vi "FGEN_OPEN.vi"(8 "error in":errorcluster caption="error in (no error)", 10 "channel parameters":T3(array[cluster])=[{"channel name"="0", "waveform"=5, "frequency"=1000000.0, "amplitude"=1.0, "start phase"=0.0, "dc offset"=-0.05, "duty cycle high"=50.0, "impedance"=0, "load impedance"=-1.0}] {"waveform" items=["Sine", "Square", "Triangle", "Ramp Up", "Ramp Down", "DC", "Noise", "User"]; "impedance" items=["50 ohms", "75 ohms"]}, 11 "resource name":refnum<k15>="PXI1Slot2") -> (0 "error out":errorcluster, 3 "Instrument Handle Out":refnum<k15>)   [LabVIEW 2013]
doc: "Configures and runs National Instruments signal generators using NI-FGEN in Standard Function output mode.\n\nYou must place at least two NI-FGEN Express (Standard Functions) VIs on the block diagram for successful function generation. Select <B>Start generation</B> for the Generation Mode in the first Express VI to start the continuous function generation. Select <B>Stop generation</B> for the Generation Mode in the final Express VI to abort function generation and close the NI-FGEN device handle.\n--------------------\n\nThis Express VI is configured as follows:\n\nDevice: PXI1Slot2 (PXI-5402)\nChannel 0\n - Waveform: DC\n - Frequency: 1MHz\n - Amplitude: 1Vpk\n - Start phase: 0 degrees\n - DC offset: -50mV\n - Output impedance: 50 Ohm\n - Load impedance: Matching\nReference clock source: Internal"
uses:
  <instrlib>/niFgen/niFgen.llb/niFgen Waveform Type.ctl
  <instrlib>/niFgen/niFgen.llb/niFgen Output Impedance.ctl
  <instrlib>/niFgen/niFgen.llb/niFgen Output Mode.ctl
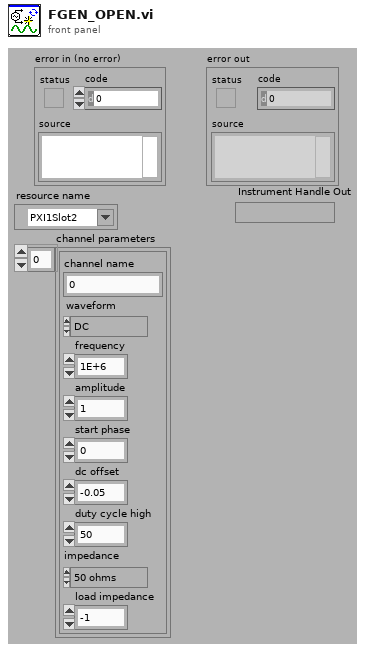
[diagram p1: front panel]
types:
  T1 = typedef "niFgen Waveform Type.ctl" = i32
  T2 = typedef "niFgen Output Impedance.ctl" = i32
  T3 = cluster{"channel name":string, "waveform":T1, "frequency":dbl, "amplitude":dbl, "start phase":dbl, "dc offset":dbl, "duty cycle high":dbl, "impedance":T2, "load impedance":dbl}[]
  T4 = typedef "niFgen Output Mode.ctl" = u32
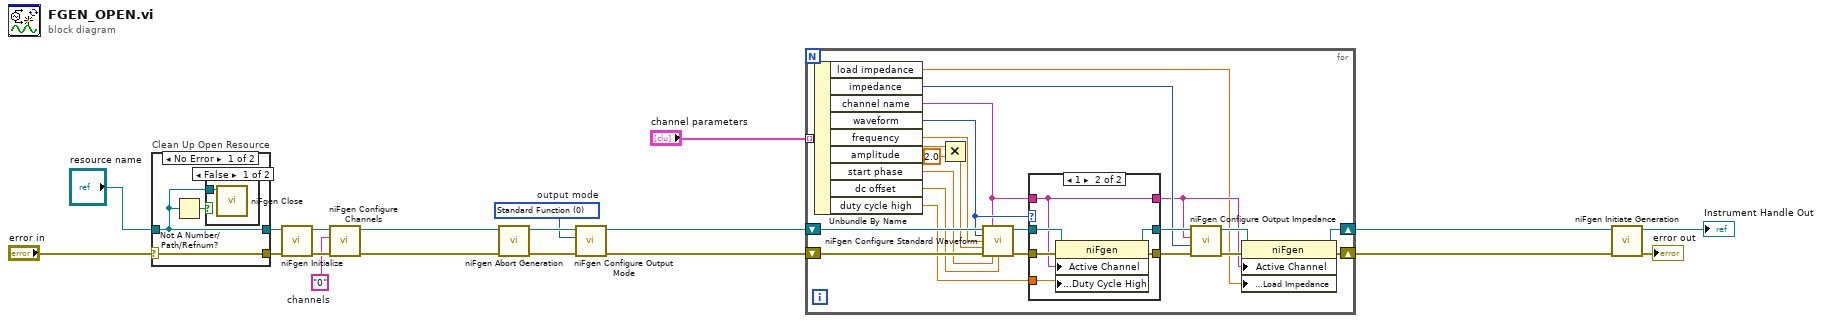
[diagram p0: block diagram]
diagram:
  w7 = T4 0 items=["Standard Function", "Frequency List", "Arbitrary Waveform", "Arbitrary Sequence", "Script"]  # output mode
  w12 = "0"  # channels
  n1 = case "Clean Up Open Resource" shown="No Error" "error in" {
    selector: "error in" -> [w21 w24]
    tunnel: "resource name" -> [w20 w25]
    tunnel: [w21 w24] -> w17
    tunnel: [w20 w25] -> w18
    frame No Error {
      n2 = Not A Number/Path/Refnum?(number/path/refnum=w20) -> (NaN/Path/Refnum?=w22:bool)
      n3 = case shown="False" w22 {
        tunnel: w20 -> [w23 _]
        frame False {
          n4 = call <instrlib>:"niFgen Close.vi"("Instrument Handle"=w23) -> ()  [unwired: 10 in, 1 out]
        }
        frame True {
        }
      }
    }
    frame Error {
    }
  }
  n5 = call <instrlib>:"niFgen Initialize.vi"("error in (no error)"=w17, "Resource Name"=w18) -> ("error out"=w15:errorcluster, "Instrument Handle Out"=w14:refnum<k15>)  [unwired: 8 in]
  n6 = call <instrlib>:"niFgen Configure Channels.vi"("error in (no error)"=w15, "Channels"=w12, "Instrument Handle"=w14) -> ("error out"=w13:errorcluster, "Instrument Handle Out"=w11:refnum<k15>)  [unwired: 7 in]
  n7 = call <instrlib>:"niFgen Abort Generation.vi"("error in (no error)"=w13, "Instrument Handle"=w11) -> ("error out"=w9:errorcluster, "Instrument Handle Out"=w8:refnum<k15>)  [unwired: 8 in]
  n8 = call <instrlib>:"niFgen Configure Output Mode.vi"("error in (no error)"=w9, "Output Mode (default: 0=Standard Function)"=w7, "Instrument Handle"=w8) -> ("error out"=w5:errorcluster, "Instrument Handle Out"=w6:refnum<k15>)  [unwired: 6 in]
  n9 = for {
    tunnel: "channel parameters" -> [w42] mode=indexing
    shift-right: [w29] -> w2
    shift-left: w6 -> [w44]
    shift-right: [w30] -> w10
    shift-left: w5 -> [w43]
    n10 = Unbundle By Name(w42) -> ("load impedance"=w31:dbl, "impedance"=w35:T2, "channel name"=w36:string, "waveform"=w41:T1, "frequency"=w40:dbl, "amplitude"=w28:dbl, "start phase"=w39:dbl, "dc offset"=w38:dbl, "duty cycle high"=w37:dbl)
    n11 = Multiply(x=w28, y=2.0 ("convert Vpk to Vpk-pk")) -> (x*y=w27:dbl)
    n12 = call <instrlib>:"niFgen Configure Standard Waveform.vi"("Instrument Handle"=w44, "Channel Name"=w36, "Waveform"=w41, "Frequency"=w40, "Amplitude"=w27, "error in (no error)"=w43, "Start Phase"=w39, "DC Offset"=w38) -> ("Instrument Handle Out"=w47:refnum<k15>, "error out"=w48:errorcluster)  [unwired: 6 in]
    n13 = case "waveformCase" shown="1" w41 {
      tunnel: [w50 w57] -> w46
      tunnel: [w51 w56] -> w45
      tunnel: w48 -> [w50 w55]
      tunnel: w47 -> [w51 w54]
      tunnel: w37 -> [_ w53]
      tunnel: w36 -> [w49 w52]
      tunnel: [w49 w52] -> w32
      frame Default {
      }
      frame 1 {
        n14 = property class="niFgen"(reference=w54, error in=w55, "Active Channel"=w52, "Standard Function Output:Duty Cycle High"=w53) -> (reference out=w56:refnum<k15>, error out=w57:errorcluster)
      }
    }
    n15 = call <instrlib>:"niFgen Configure Output Impedance.vi"("error in (no error)"=w46, "Impedance (default: 0=50 ohms)"=w35, "Channel Name"=w32, "Instrument Handle"=w45) -> ("error out"=w34:errorcluster, "Instrument Handle Out"=w33:refnum<k15>)  [unwired: 6 in]
    n16 = property class="niFgen"(reference=w33, error in=w34, "Active Channel"=w32, "Output Attributes:Load Impedance"=w31) -> (reference out=w29:refnum<k15>, error out=w30:errorcluster)
  }
  n17 = call <instrlib>:"niFgen Initiate Generation.vi"("error in (no error)"=w10, "Instrument Handle"=w2) -> ("error out"=→"error out":errorcluster, "Instrument Handle Out"=→"Instrument Handle Out":refnum<k15>)  [unwired: 8 in]
